vi "Query Output.vi"(8 "error in (no error)":errorcluster, 11 "336XX in":refnum<class "336XX.lvclass">) -> (0 "error out":errorcluster, 2 "Output":bool, 3 "336XX out":refnum<class "336XX.lvclass">)   [LabVIEW 2019, in "336XX.lvlib" / "336XX.lvclass"]
uses:
  Library/336XX.lvclass
  C:/Users/Public/Documents/Development/builds/Instruments/FunctionGenerator.lvlibp/Library/FunctionGenerator.lvclass
  builds/Instruments/FunctionGenerator.lvlibp/Accessors/Read Active Channel.vi
  builds/Engine/Engine.lvlibp/Project/Engine.lvclass
  C:/Users/Public/Documents/Development/builds/Engine/Engine.lvlibp/Project/Engine.lvclass
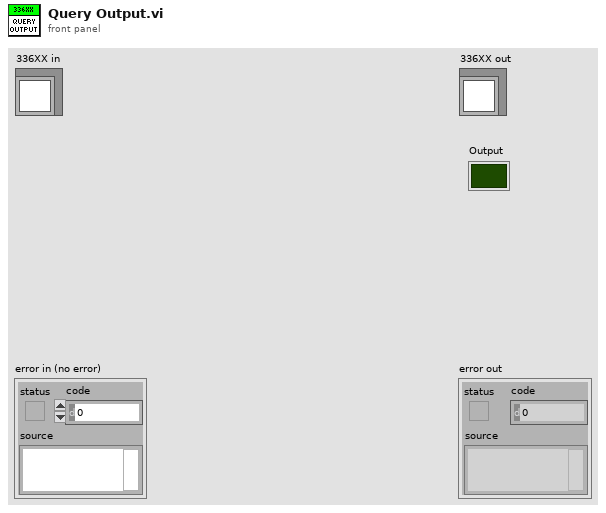
[diagram p1: front panel]
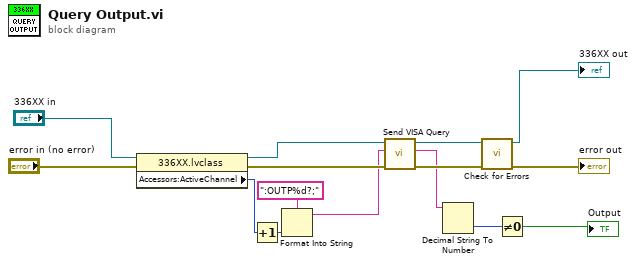
[diagram p0: block diagram]
diagram:
  n1 = property class="336XX.lvclass"(reference="336XX in", error in="error in (no error)") -> (reference out=w13:refnum<class "336XX.lvclass">, error out=w12:errorcluster, "Accessors:ActiveChannel"=w11:i32)
  n2 = Increment(x=w11) -> (x+1=w1:i32)
  n3 = Format Into String(format string=":OUTP%d?;", w1) -> (resulting string=w9:string)  [unwired: 2 in, 1 out]
  n4 = call "Send VISA Query.vi"("error in (no error)"=w12, "Command"=w9, "336XX in"=w13) -> ("error out"=w8:errorcluster, "Response"=w7:string, "336XX out"=w3:refnum<class "336XX.lvclass">)  [unwired: 6 in]
  n5 = Decimal String To Number(string=w7) -> (number=w6:i32)  [unwired: 2 in, 1 out]
  n6 = call "Check for Errors.vi"("error in"=w8, "Engine in"=w3) -> ("error out"=→"error out":errorcluster, "Engine out"=→"336XX out":refnum<class "336XX.lvclass">)  [unwired: 8 in]
  n7 = Not Equal To 0?(x=w6) -> (x != 0?=→"Output":bool)
